vi "2D Heat PDE Solver (Rect Domain).vi"(0 "PDE in":refnum<class "NI_PDE.lvclass">, 11 "error in (no error)":errorcluster) -> (4 "PDE out":refnum<class "NI_PDE.lvclass">, 6 "U(t, x, y)":dbl[][][](array[numeric]), 15 "error out":errorcluster)   [LabVIEW 2020, in "NI_PDE.lvlib"]
doc: "Solves a partial differential equation. You must manually select the polymorphic instance to use."
uses:
  <vilib>/gmath/NI_PDE.lvlib
  <vilib>/gmath/pde.llb/PDEClass/NI_PDE.lvclass
  <vilib>/gmath/pde.llb/ICClass/IC_2D_Numeric/NI_IC_2D_Numeric.lvclass
  e:/builds/penguin/labview/branches/2020/dev/dist/vi.lib/gmath/pde.llb/ICClass/NI_IC.lvclass
  <vilib>/gmath/pde.llb/PDEClass/PDE_Heat_2D/NI_PDE_Heat_2D.lvclass
  e:/builds/penguin/labview/branches/2020/dev/dist/vi.lib/gmath/pde.llb/PDEClass/NI_PDE.lvclass
  <vilib>/gmath/pde.llb/RHSClass/RHS_3D_Numeric/NI_RHS_3D_Numeric.lvclass
  e:/builds/penguin/labview/branches/2020/dev/dist/vi.lib/gmath/pde.llb/RHSClass/NI_RHS.lvclass
  <vilib>/gmath/pde.llb/BCClass/BC_Evolut_2D_Numeric/NI_BC_Evolut_2D_Numeric.lvclass
  e:/builds/penguin/labview/branches/2020/dev/dist/vi.lib/gmath/pde.llb/BCClass/NI_BC.lvclass
  <vilib>/gmath/pde.llb/DomainClass/Domain_Evolut_2D_Rect/NI_Domain_Evolut_2D_Rect.lvclass
  e:/builds/penguin/labview/branches/2020/dev/dist/vi.lib/gmath/pde.llb/DomainClass/NI_Domain.lvclass
  <vilib>/gmath/pde.llb/DomainClass/Domain_Evolut_2D_Rect/Domain Data.ctl
  <vilib>/gmath/pde.llb/PDEClass/PDE_2ndOrder_ConstPara/Para Data.ctl
  <vilib>/gmath/pde.llb/PDEClass/PDE Data_Class.ctl
  <vilib>/gmath/pde.llb/RHSClass/NI_RHS.lvclass
  <vilib>/gmath/pde.llb/DomainClass/NI_Domain.lvclass
  <vilib>/gmath/pde.llb/BCClass/NI_BC.lvclass
  <vilib>/gmath/pde.llb/ICClass/NI_IC.lvclass
  <vilib>/gmath/pde.llb/ICClass/IC_2D_Numeric/IC Data.ctl
  <vilib>/gmath/pde.llb/Common/PDE_IC Type.ctl
  <vilib>/gmath/pde.llb/BCClass/BC_Evolut_2D_Numeric/BC Data.ctl
  <vilib>/gmath/pde.llb/Common/PDE_BC Type.ctl
  <vilib>/gmath/pde.llb/Common/PDE_BC Position 2D.ctl
  <vilib>/gmath/pde.llb/PDEClass/PDE_2ndOrder_ConstPara/NI_PDE_2ndOrder_ConstPara.lvclass
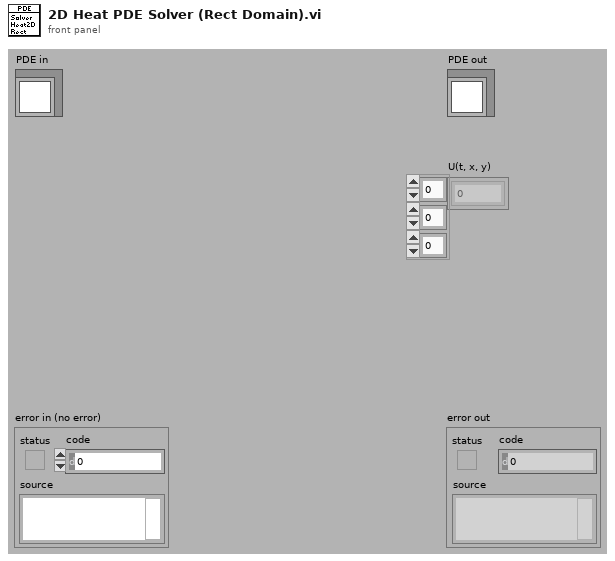
[diagram p1: front panel]
types:
  T1 = typedef "NI_PDE.lvlib/NI_IC_2D_Numeric.lvclass/IC Data.ctl" = cluster{"type":T2, "H":dbl[][]}
  T2 = typedef "NI_PDE.lvlib/PDE_IC Type.ctl" = i32
  T3 = typedef "NI_PDE.lvlib/NI_PDE.lvclass/PDE Data_Class.ctl" = cluster{"PDE":refnum<class "NI_PDE.lvclass">, "RHS":refnum<class "NI_RHS.lvclass">, "Domain":refnum<class "NI_Domain.lvclass">, "BC":refnum<class "NI_BC.lvclass">, "IC":refnum<class "NI_IC.lvclass">}
  T4 = typedef "NI_PDE.lvlib/NI_PDE_2ndOrder_ConstPara.lvclass/Para Data.ctl" = cluster{"k":dbl, "a":dbl}
  T5 = typedef "NI_PDE.lvlib/NI_Domain_Evolut_2D_Rect.lvclass/Domain Data.ctl" = cluster{"T":cluster{"initial t":dbl, "final t":dbl, "# of t-points":i32}, "X":cluster{"start x":dbl, "end x":dbl, "# of x-points":i32}, "Y":cluster{"start y":dbl, "end y":dbl, "# of y-points":i32}}
  T6 = typedef "NI_PDE.lvlib/NI_BC_Evolut_2D_Numeric.lvclass/BC Data.ctl" = cluster{"type":T7, "position":T8, "G":dbl[][]}
  T7 = typedef "NI_PDE.lvlib/PDE_BC Type.ctl" = i32
  T8 = typedef "NI_PDE.lvlib/PDE_BC Position 2D.ctl" = i32
  T9 = typedef "NI_PDE.lvlib/NI_PDE.lvclass/PDE Data_Variant.ctl" = cluster{"parameter":variant, "RHS":variant, "domain":variant, "BC Array":variant[], "IC Array":variant[]}
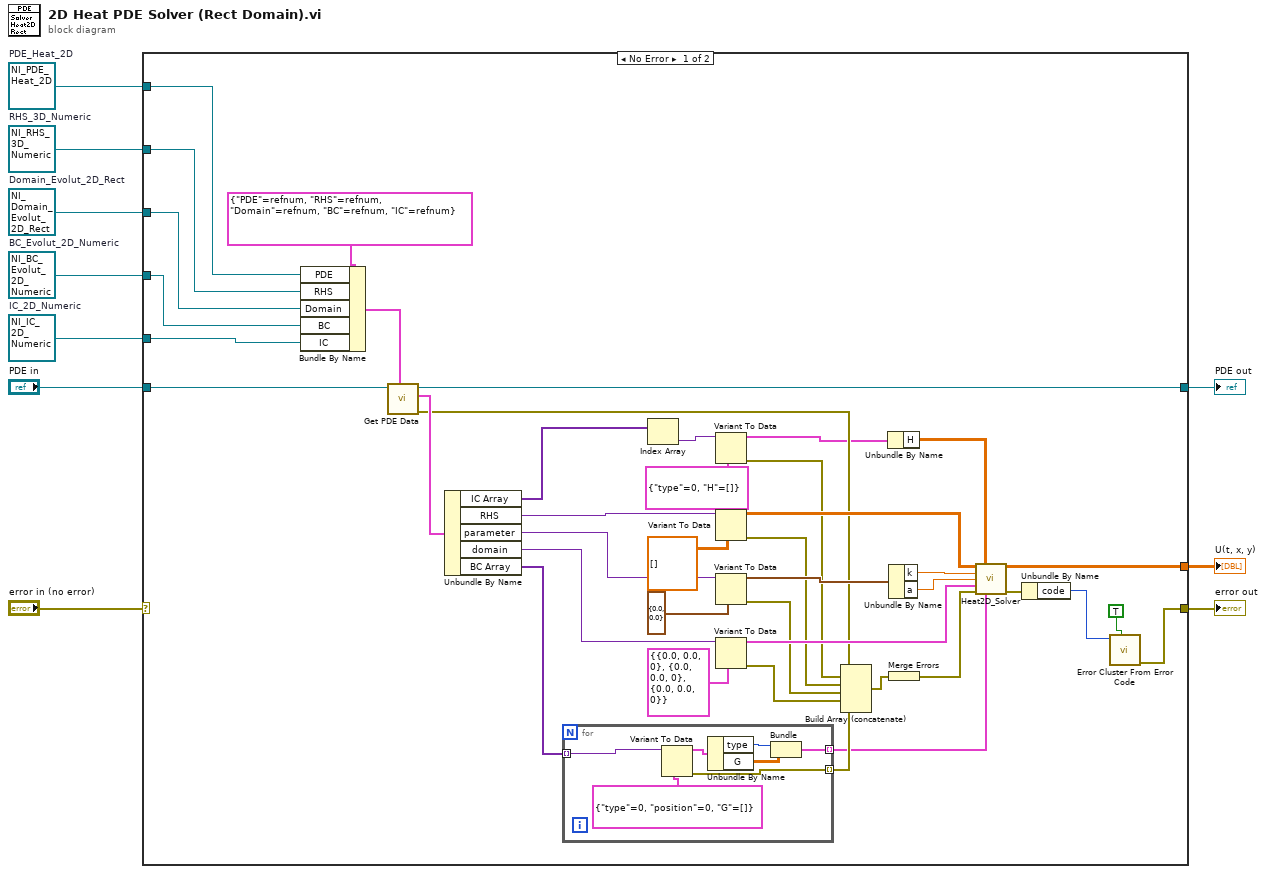
[diagram p0: block diagram]
diagram:
  w3 = refnum<class "NI_Domain_Evolut_2D_Rect.lvclass"> refnum  # Domain_Evolut_2D_Rect
  w4 = refnum<class "NI_BC_Evolut_2D_Numeric.lvclass"> refnum  # BC_Evolut_2D_Numeric
  w2 = refnum<class "NI_RHS_3D_Numeric.lvclass"> refnum  # RHS_3D_Numeric
  w1 = refnum<class "NI_PDE_Heat_2D.lvclass"> refnum  # PDE_Heat_2D
  w5 = refnum<class "NI_IC_2D_Numeric.lvclass"> refnum  # IC_2D_Numeric
  n1 = case shown="No Error" "error in (no error)" {
    selector: "error in (no error)" -> [_ w59]
    tunnel: [w51 _] -> w7
    tunnel: "PDE in" -> [w31 w60]
    tunnel: [w30 w60] -> w8
    tunnel: [w47 w59] -> w6
    tunnel: w1 -> [w23 _]
    tunnel: w3 -> [w21 _]
    tunnel: w4 -> [w20 _]
    tunnel: w2 -> [w22 _]
    tunnel: w5 -> [w18 _]
    frame No Error {
      n2 = Bundle By Name(cluster=T3 {"PDE"=refnum, "RHS"=refnum, "Domain"=refnum, "BC"=refnum, "IC"=refnum} ("target class"), "PDE"=w23, "RHS"=w22, "Domain"=w21, "BC"=w20, "IC"=w18) -> (w19:T3)
      n3 = call <vilib>:"Get PDE Data.vi"("target class"=w19, "PDE in"=w31) -> ("error out"=w14:errorcluster, "PDE data"=w29:T9, "PDE out"=w30:refnum<class "NI_PDE.lvclass">)  [unwired: 3 in, 4 out]
      n4 = Unbundle By Name(w29) -> ("IC Array"=w17:variant[], "RHS"=w27:variant, "parameter"=w28:variant, "domain"=w26:variant, "BC Array"=w25:variant[])
      n5 = for {
        tunnel: w25 -> [w57] mode=indexing
        tunnel: [w58] -> w35 mode=indexing
        tunnel: [w53] -> w32 mode=indexing
        n6 = Variant To Data(type=T6 {"type"=0, "position"=0, "G"=[]} ("BC data"), Variant=w57) -> (data=w56:T6, error out=w58:errorcluster)  [unwired: 1 in]
        n7 = Unbundle By Name(w56) -> ("type"=w55:T7, "G"=w54:dbl[][])
        n8 = Bundle("type"=w55, "G"=w54) -> (w53:cluster{"type":T7, "G":dbl[][]})  [unwired: 1 out]
      }
      n9 = Index Array(array=w17) -> (element=w16:variant)  [unwired: 1 in]
      n10 = Variant To Data(type=T1 {"type"=0, "H"=[]} ("Initial Value"), Variant=w16) -> (data=w12:T1, error out=w13:errorcluster)  [unwired: 1 in]
      n11 = Variant To Data(type=dbl[][][] [] ("F(x, y)"), Variant=w27) -> (data=w39:dbl[][][], error out=w38:errorcluster)  [unwired: 1 in]
      n12 = Variant To Data(type=T4 {"k"=0.0, "a"=0.0} ("para data"), Variant=w28) -> (data=w43:T4, error out=w37:errorcluster)  [unwired: 1 in]
      n13 = Variant To Data(type=T5 {"T"={"initial t"=0.0, "final t"=0.0, "# of t-points"=0}, "X"={"start x"=0.0, "end x"=0.0, "# of x-points"=0}, "Y"={"start y"=0.0, "end y"=0.0, "# of y-points"=0}} ("domain data"), Variant=w26) -> (data=w45:T5, error out=w36:errorcluster)  [unwired: 1 in]
      n14 = Build Array (concatenate)(w14, w13, w38, w37, w36, w35) -> (w34:errorcluster[])
      n15 = Unbundle By Name(w12) -> ("H"=w11:dbl[][])
      n16 = Unbundle By Name(w43) -> ("k"=w42:dbl, "a"=w41:dbl)
      n17 = Merge Errors(w34) -> (w33:errorcluster)
      n18 = call <vilib>:"Heat2D_Solver.vi"("F(t, x, y)"=w39, "Initial Value"=w11, "k"=w42, "a"=w41, "Domain"=w45, "error in (no error)"=w33, "Boundary Condition"=w32) -> ("U(t, x, y)"=w51:dbl[][][], "error out"=w48:errorcluster)  [unwired: 7 out]
      n19 = Unbundle By Name(w48) -> ("code"=w50:i32)
      n20 = call <vilib>:"Error Cluster From Error Code.vi"("show call chain? (False)"=TRUE, "error code (0)"=w50) -> ("error out"=w47:errorcluster)  [unwired: 1 in, 6 out]
    }
    frame Error {
    }
  }
  "U(t, x, y)" <- w7
  "error out" <- w6
  "PDE out" <- w8
